vi "Move Home.vi"(8 "error in (no error)":errorcluster, 11 "Stage Controller in":refnum<class "Stage Controller.lvclass">) -> (0 "error out":errorcluster, 3 "Stage Controller out":refnum<class "Stage Controller.lvclass">)   [LabVIEW 2018, in "Stage Controller.lvlib" / "Stage Controller.lvclass"]
uses:
  Stage Controller.lvclass
  Stage Controller.lvclass/Stage Controller.ctl
  Ti2/ti2lv/ti2lv.lvlib
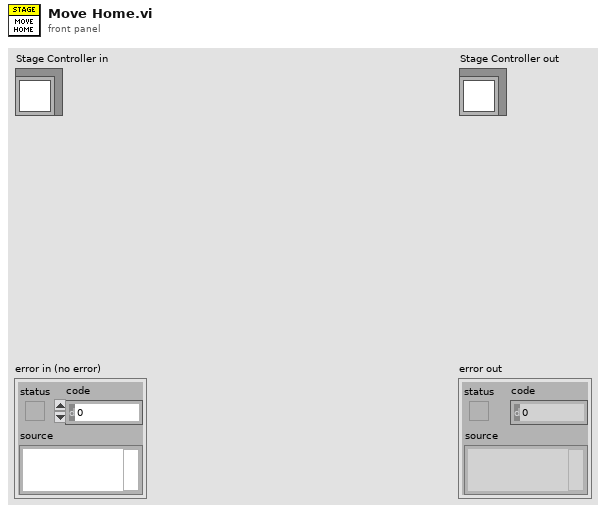
[diagram p1: front panel]
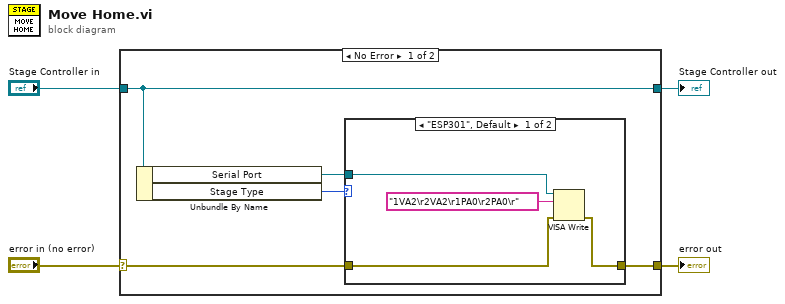
[diagram p0: block diagram]
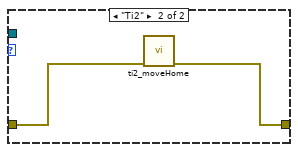
[diagram p2: hidden frame]
diagram:
  n1 = case shown="No Error" "error in (no error)" {
    selector: "error in (no error)" -> [w8 w17]
    tunnel: [w7 w17] -> w3
    tunnel: [w9 w16] -> w1
    tunnel: "Stage Controller in" -> [w9 w16]
    frame No Error {
      n2 = Unbundle By Name(w9) -> ("Serial Port"=w5:refnum<visa-resource-name>, "Stage Type"=w6:enum16{"ESP301", "Ti2"})
      n3 = case shown="\"ESP301\", Default" w6 {
        tunnel: w8 -> [w10 w15]
        tunnel: [w11 w14] -> w7
        tunnel: w5 -> [w12 _]
        frame "ESP301", Default {
          n4 = VISA Write(VISA resource name=w12, write buffer="1VA2\r2VA2\r1PA0\r2PA0\r", error in (no error)=w10) -> (error out=w11:errorcluster)  [unwired: 2 out]
        }
        frame "Ti2" {
          n5 = call "ti2_moveHome.vi"("error in (no error)"=w15) -> ("error out"=w14:errorcluster)  [unwired: 10 in]
        }
      }
    }
    frame Error {
    }
  }
  "error out" <- w3
  "Stage Controller out" <- w1
